vi "test_NonReentrantMeasurement_MultipleMeasureCalls_ExecuteInSequence.vi"(8 "error in":errorcluster) -> (0 "error out":errorcluster, 2 "result":string, 3 "pass":bool)   [LabVIEW 2021, in "MeasurementServerTests.lvlib" / "Measurement Service Tests.lvlib"]
uses:
  Measurement Service Tests.lvlib
  Runtime/Measurements/Helpers/TypeDefs/Measurement Server User Settings.ctl
  Runtime/Measurements/Helpers/TypeDefs/Stop Server User Event.ctl
  Runtime/Measurements/Helpers/TypeDefs/Measurement Service Version.ctl
  Continuous Counting Client/controls/Measurement Configuration.ctl
  Continuous Counting Measurement/Continuous Counting Measurement.lvclass
  Runtime/Measurements/NI Measurement Plug-In SDK.lvlib
  Continuous Counting Client/Continuous Counting Client.lvlib
  MeasurementServerTests.lvlib
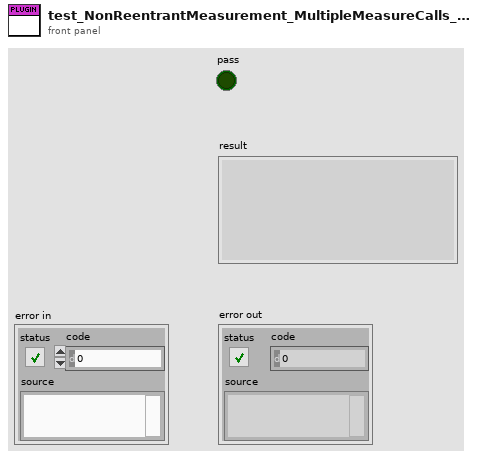
[diagram p1: front panel]
types:
  T1 = typedef "NI Measurement Plug-In SDK.lvlib/Measurement Service Version.ctl" = enum16{"V1", "V2"}
  T2 = typedef "NI Measurement Plug-In SDK.lvlib/Measurement Server User Settings.ctl" = cluster{"stop server":T3, "measurement service versions":T1[]}
  T3 = typedef "NI Measurement Plug-In SDK.lvlib/Stop Server User Event.ctl" = refnum<user-event>
  T4 = typedef "grpc-lvsupport-release.lvlib/grpcId.ctl" = u64
  T5 = typedef "MeasurementServerTests.lvlib/Measurement Service Tests.lvlib/Continuous Counting Client.lvlib/Measurement Configuration.ctl" = cluster{"ms update interval":u32}
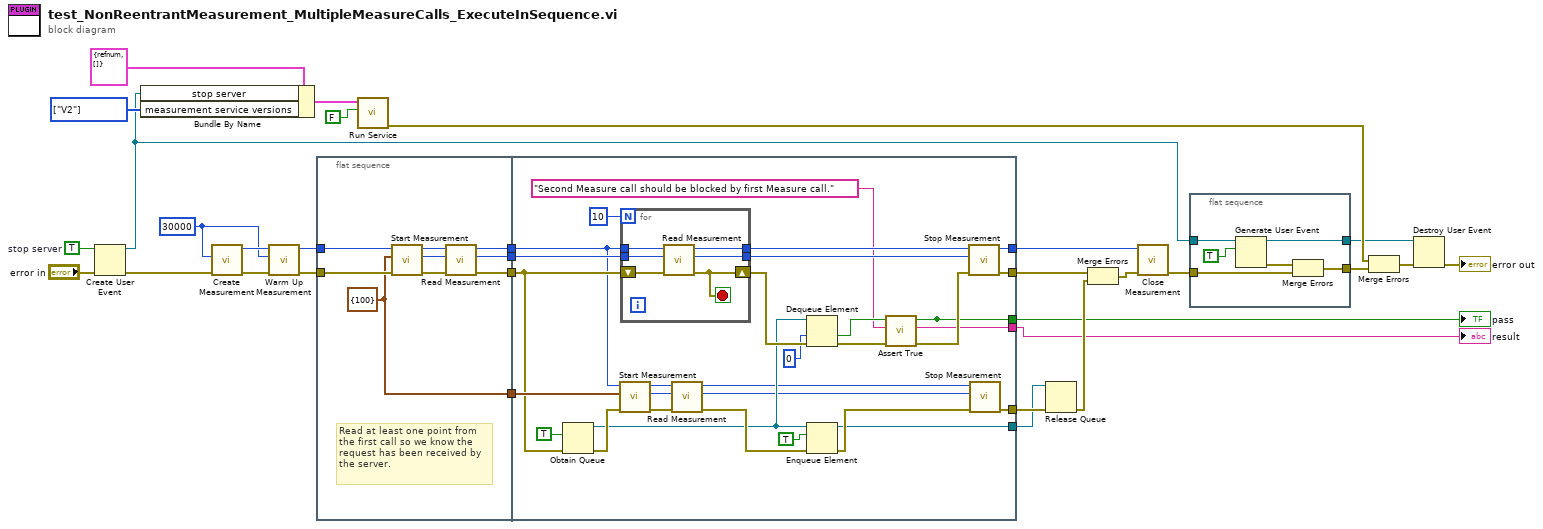
[diagram p0: block diagram]
diagram:
  w5 = 30000 ("ms timeout")
  w29 = TRUE  # stop server
  w30 = T1[] [enum."V2"] items=["V1", "V2"] ("measurement service versions")
  n1 = Create User Event(user event datatype=w29, error in="error in") -> (user event=w24:refnum<user-event>, error out=w25:errorcluster)
  n2 = Bundle By Name(cluster=T2 {"stop server"=refnum, "measurement service versions"=[]} ("server settings"), "stop server"=w24, "measurement service versions"=w30) -> (w28:T2)
  n3 = call "Create Measurement.vi"("error in"=w25, "ms timeout"=w5) -> ("error out"=w9:errorcluster, "gRPCid out"=w6:T4)  [unwired: 8 in]
  n4 = call "Warm Up Measurement.vi"("error in"=w9, "timeout (ms)"=w5, "gRPC ID"=w6) -> ("error out"=w8:errorcluster, "gRPC ID out"=w7:T4)  [unwired: 7 in]
  n5 = flat-sequence {
    tunnel: w8 -> [w40]
    tunnel: w7 -> [w39]
    tunnel: [w36] -> w20
    tunnel: [w35] -> w19
    tunnel: [w32] -> w18
    tunnel: [w33] -> w17
    tunnel: [w64] -> w14
    tunnel: w20 -> [w61]
    tunnel: w19 -> [w41]
    tunnel: w18 -> [w70]
    tunnel: w17 -> [w65]
    tunnel: [w50] -> w16
    tunnel: [w45] -> w15
    tunnel: [w44] -> w12
    tunnel: [w42] -> _
    tunnel: [w43] -> w11
    tunnel: [w42] -> w10
    frame #0 {
      w33 = T5 {"ms update interval"=100} ("measurement configuration")
      # "Read at least one point from\nthe first call so we know the\nrequest has been received by\nthe server."
      n6 = call "Start Measurement.vi"("error in"=w40, "measurement configuration"=w33, "gRPCid in"=w39) -> ("error out"=w37:errorcluster, "call id"=w34:T4, "gRPCid out"=w38:T4)  [unwired: 6 in]
      n7 = call "Read Measurement.vi"("error in"=w37, "call id in"=w34, "gRPCid in"=w38) -> ("error out"=w36:errorcluster, "call id out"=w32:T4, "gRPCid out"=w35:T4)  [unwired: 4 in, 2 out]
    }
    frame #1 {
      n8 = Obtain Queue(element data type=TRUE, error in (no error)=w61) -> (queue out=w55:refnum<queue>, error out=w59:errorcluster)  [unwired: 3 in, 1 out]
      n9 = call "Start Measurement.vi"("error in"=w59, "measurement configuration"=w65, "gRPCid in"=w41) -> ("error out"=w68:errorcluster, "call id"=w66:T4, "gRPCid out"=w67:T4)  [unwired: 6 in]
      n10 = for {
        N: 10 -> [_]
        shift-right: [w72] -> w56
        shift-left: w61 -> [w76]
        tunnel: w41 -> [w75]
        tunnel: w70 -> [w74]
        tunnel: [w73] -> w63
        tunnel: [w71] -> w62
        stop <- w72 stop-if-true
        n11 = call "Read Measurement.vi"("error in"=w76, "call id in"=w74, "gRPCid in"=w75) -> ("error out"=w72:errorcluster, "call id out"=w71:T4, "gRPCid out"=w73:T4)  [unwired: 4 in, 2 out]
      }
      n12 = call "Read Measurement.vi"("error in"=w68, "call id in"=w66, "gRPCid in"=w67) -> ("error out"=w58:errorcluster, "call id out"=w52:T4, "gRPCid out"=w53:T4)  [unwired: 4 in, 2 out]
      n13 = Dequeue Element(queue=w55, timeout in ms (-1)=0, error in (no error)=w56) -> (timed out?=w47:bool, error out=w49:errorcluster)  [unwired: 2 out]
      n14 = Enqueue Element(queue=w55, element=TRUE, error in (no error)=w58) -> (queue out=w45:refnum<queue>, error out=w51:errorcluster)  [unwired: 1 in, 1 out]
      n15 = call "Assert True.vi"("error in"=w49, "failure message"="Second Measure call should be blocked by first Measure call.", "condition"=w47) -> ("error out"=w48:errorcluster, "message"=w43:string, "pass"=w42:bool)  [unwired: 6 in]
      n16 = call "Stop Measurement.vi"("error in"=w48, "call id"=w62, "gRPCid in"=w63) -> ("error out"=w64:errorcluster, "gRPCid out"=w44:T4)  [unwired: 7 in]
      n17 = call "Stop Measurement.vi"("error in"=w51, "call id"=w52, "gRPCid in"=w53) -> ("error out"=w50:errorcluster)  [unwired: 7 in, 1 out]
    }
  }
  n18 = call "Run Service.vi"("reentrant"=FALSE, "server settings"=w28) -> ("error out"=w23:errorcluster)  [unwired: 9 in]
  n19 = Release Queue(queue=w15, error in (no error)=w16) -> (error out=w13:errorcluster)  [unwired: 1 in, 2 out]
  n20 = Merge Errors(w14, w13) -> (w26:errorcluster)
  n21 = call "Close Measurement.vi"("error in"=w26, "gRPCid in"=w12) -> ("error out"=w22:errorcluster)  [unwired: 9 in]
  n22 = flat-sequence {
    tunnel: w24 -> [w81]
    tunnel: [w80] -> w2
    tunnel: [w79] -> w4
    tunnel: w22 -> [w78]
    frame #0 {
      n23 = Generate User Event(user event=w81, event data cluster=TRUE ("event data")) -> (user event out=w80:refnum<user-event>, error out=w82:errorcluster)  [unwired: 2 in]
      n24 = Merge Errors(w82, w78) -> (w79:errorcluster)
    }
  }
  n25 = Merge Errors(w23, w4) -> (w3:errorcluster)
  n26 = Destroy User Event(user event=w2, error in=w3) -> (error out=→"error out":errorcluster)
  "pass" <- w10
  "result" <- w11
